vi "createTest.vi"(4 "id":u32, 6 "humidity":string, 7 "temp":string, 8 "error in (no error)":errorcluster, 9 "TestName":string, 10 "report ref":refnum<k20>, 11 "DOM document":refnum<k20>) -> (0 "error out":errorcluster, 1 "dup Report ref":refnum<k20>, 2 "test ref":refnum<k20>, 3 "dup DOM document":refnum<k20>)   [LabVIEW 2013]
uses:
  <resource>/objmgr/DOMUserDefRef.rc
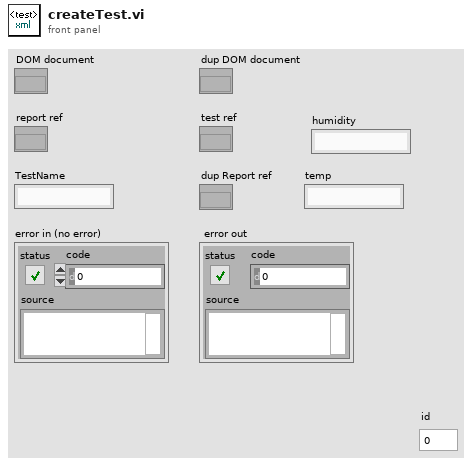
[diagram p1: front panel]
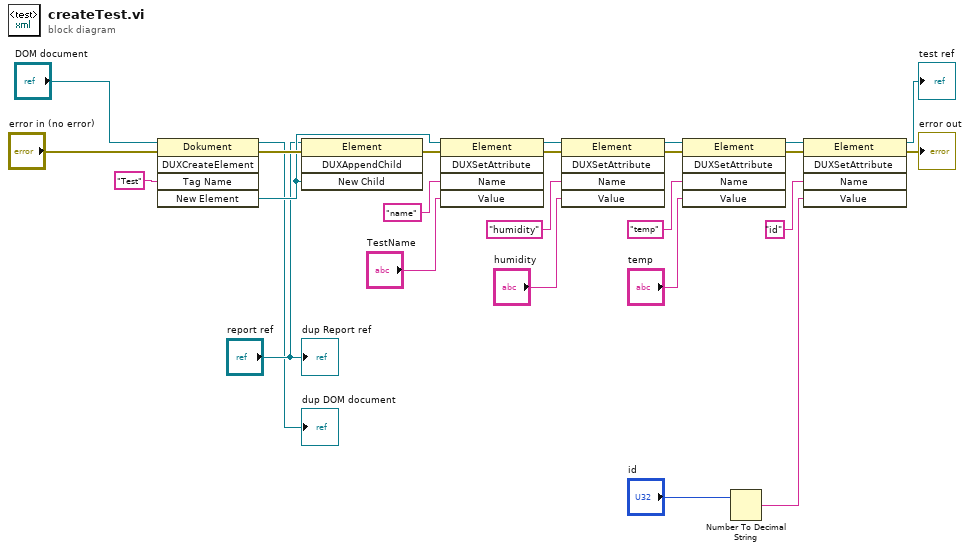
[diagram p0: block diagram]
diagram:
  n1 = invoke class="Dokument" method="DUXCreateElement"(reference="DOM document", error in="error in (no error)", "Tag Name"="Test" ("Qualified Name")) -> (reference out=→"dup DOM document":refnum<k20>, error out=w21:errorcluster, "New Element"=w18:refnum<k20>)  [unwired: 2 in, 2 out]
  n2 = invoke class="Element" method="DUXAppendChild"(reference="report ref", error in=w21, "New Child"=w18) -> (error out=w20:errorcluster)  [unwired: 1 in, 3 out]
  n3 = invoke class="Element" method="DUXSetAttribute"(reference=w18, error in=w20, "Name"="name" ("Tag Name"), "Value"="TestName") -> (reference out=w13:refnum<k20>, error out=w12:errorcluster)  [unwired: 1 in, 3 out]
  n4 = invoke class="Element" method="DUXSetAttribute"(reference=w13, error in=w12, "Name"="humidity" ("Tag Name"), "Value"="humidity") -> (reference out=w9:refnum<k20>, error out=w8:errorcluster)  [unwired: 1 in, 3 out]
  n5 = invoke class="Element" method="DUXSetAttribute"(reference=w9, error in=w8, "Name"="temp" ("Tag Name"), "Value"="temp") -> (reference out=w7:refnum<k20>, error out=w6:errorcluster)  [unwired: 1 in, 3 out]
  n6 = Number To Decimal String(number="id") -> (decimal integer string=w4:string)  [unwired: 1 in]
  n7 = invoke class="Element" method="DUXSetAttribute"(reference=w7, error in=w6, "Name"="id", "Value"=w4) -> (reference out=→"test ref":refnum<k20>, error out=→"error out":errorcluster)  [unwired: 1 in, 3 out]
  "dup Report ref" <- "report ref"
